vi "Build DashBoard Data.vi"(11 "Dashboard Enables":T3={"Analog Module 1"=[TRUE, TRUE, TRUE, TRUE, TRUE, TRUE, TRUE, TRUE], "Analog Module 2"=[FALSE, FALSE, FALSE, FALSE, FALSE, FALSE, FALSE, FALSE], "Digital Module 1"=TRUE, "Digital Module 2"=FALSE, "Solenoid Module"=TRUE}) -> ()   [LabVIEW 2012]
doc: "This VI builds data and sends it back to the dashboard PC program. By default it sends back the raw values for the first analog, digital, and solenoid module. Modify it to send back the data you want to view. Consider adding higher level data to the Dashboard Datatype.ctl and to this VI. Then update the Dashboard to display the data however you like.\n\nThis software is licensed. Open the labview\\readme\\WPI Robotics Library Open Source License.txt file for more information."
uses:
  DashboardEnable.ctl
  Dashboard Datatype.ctl
  <vilib>/Rock Robotics/WPI/DriverStation/WPI_DriverStationDigitalData.ctl
  <vilib>/Rock Robotics/SystemInterfaces/System/FPGA_SystemGet.vi
panel:
  out "Dashboard Data":T1
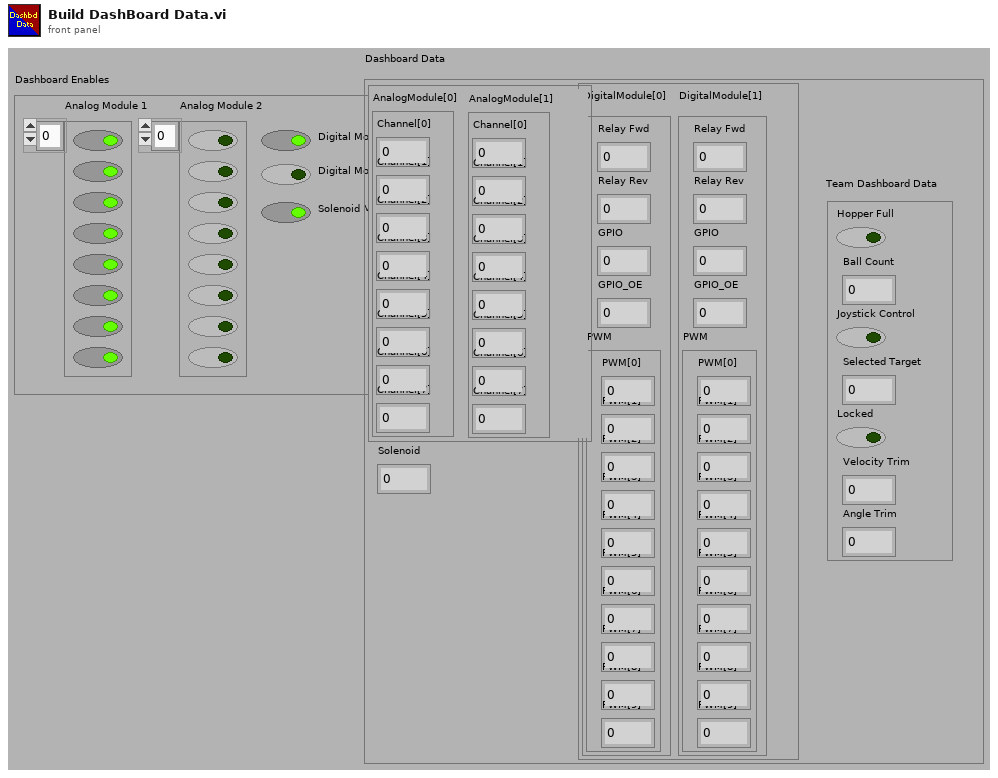
[diagram p1: front panel]
types:
  T1 = typedef "Dashboard Datatype.ctl" = cluster{cluster{"AnalogModule[0]":cluster{"Channel[0]":sgl, "Channel[1]":sgl, "Channel[2]":sgl, "Channel[3]":sgl, "Channel[4]":sgl, "Channel[5]":sgl, "Channel[6]":sgl, "Channel[7]":sgl}, "AnalogModule[1]":cluster{"Channel[0]":sgl, "Channel[1]":sgl, "Channel[2]":sgl, "Channel[3]":sgl, "Channel[4]":sgl, "Channel[5]":sgl, "Channel[6]":sgl, "Channel[7]":sgl}}, cluster{"DigitalModule[0]":T2, "DigitalModule[1]":T2}, "Solenoid":u8, "Team Dashboard Data":cluster{"Hopper Full":bool, "Ball Count":dbl, "Joystick Control":bool, "Selected Target":dbl, "Locked":bool, "Velocity Trim":dbl, "Angle Trim":dbl}}
  T2 = typedef "WPI_DriverStationDigitalData.ctl" = cluster{"Relay Fwd":u8, "Relay Rev":u8, "GPIO":u16, "GPIO_OE":u16, "PWM":cluster{"PWM[0]":u8, "PWM[1]":u8, "PWM[2]":u8, "PWM[3]":u8, "PWM[4]":u8, "PWM[5]":u8, "PWM[6]":u8, "PWM[7]":u8, "PWM[8]":u8, "PWM[9]":u8}}
  T3 = typedef "DashboardEnable.ctl" = cluster{"Analog Module 1":bool[], "Analog Module 2":bool[], "Digital Module 1":bool, "Digital Module 2":bool, "Solenoid Module":bool}
  T4 = cluster{"Hopper Full":bool, "Ball Count":dbl, "Joystick Control":bool, "Selected Target":dbl, "Locked":bool, "Velocity Trim":dbl, "Angle Trim":dbl}
  T5 = cluster{"AnalogModule[0]":cluster{"Channel[0]":sgl, "Channel[1]":sgl, "Channel[2]":sgl, "Channel[3]":sgl, "Channel[4]":sgl, "Channel[5]":sgl, "Channel[6]":sgl, "Channel[7]":sgl}, "AnalogModule[1]":cluster{"Channel[0]":sgl, "Channel[1]":sgl, "Channel[2]":sgl, "Channel[3]":sgl, "Channel[4]":sgl, "Channel[5]":sgl, "Channel[6]":sgl, "Channel[7]":sgl}}
  T6 = cluster{"Channel[0]":sgl, "Channel[1]":sgl, "Channel[2]":sgl, "Channel[3]":sgl, "Channel[4]":sgl, "Channel[5]":sgl, "Channel[6]":sgl, "Channel[7]":sgl}[]
  T7 = cluster{"Channel[0]":sgl, "Channel[1]":sgl, "Channel[2]":sgl, "Channel[3]":sgl, "Channel[4]":sgl, "Channel[5]":sgl, "Channel[6]":sgl, "Channel[7]":sgl}
  T8 = cluster{"AnalogModule[0][0]":sgl, "AnalogModule[0][1]":sgl, "AnalogModule[0][2]":sgl, "AnalogModule[0][3]":sgl, "AnalogModule[0][4]":sgl, "AnalogModule[0][5]":sgl, "AnalogModule[0][6]":sgl, "AnalogModule[0][7]":sgl}
  T9 = cluster{"[0]":cluster{"Channel[0]":sgl, "Channel[1]":sgl, "Channel[2]":sgl, "Channel[3]":sgl, "Channel[4]":sgl, "Channel[5]":sgl, "Channel[6]":sgl, "Channel[7]":sgl}, "[1]":cluster{"Channel[0]":sgl, "Channel[1]":sgl, "Channel[2]":sgl, "Channel[3]":sgl, "Channel[4]":sgl, "Channel[5]":sgl, "Channel[6]":sgl, "Channel[7]":sgl}}
  T10 = cluster{"DigitalModule[0]":T2, "DigitalModule[1]":T2}
  T11 = typedef "FPGA_DIODevRef.ctl" = cluster{"DevStatus":errorcluster, "Module":T12}
  T12 = typedef "FPGA_TypedefDigitalModule.ctl" = enum16{"Digital Module 1", "Digital Module 2"}
  T13 = cluster{"[0]":u8, "[1]":u8, "[2]":u8, "[3]":u8, "[4]":u8, "[5]":u8, "[6]":u8, "[7]":u8, "[8]":u8, "[9]":u8}
  T14 = typedef "FPGA_SolenoidDevRef.ctl" = cluster{"DevStatus":errorcluster, "Module":T15}
  T15 = typedef "FPGA_TypedefSolenoidModule.ctl" = enum16{"Solenoid Module 1", "Solenoid Module 2"}
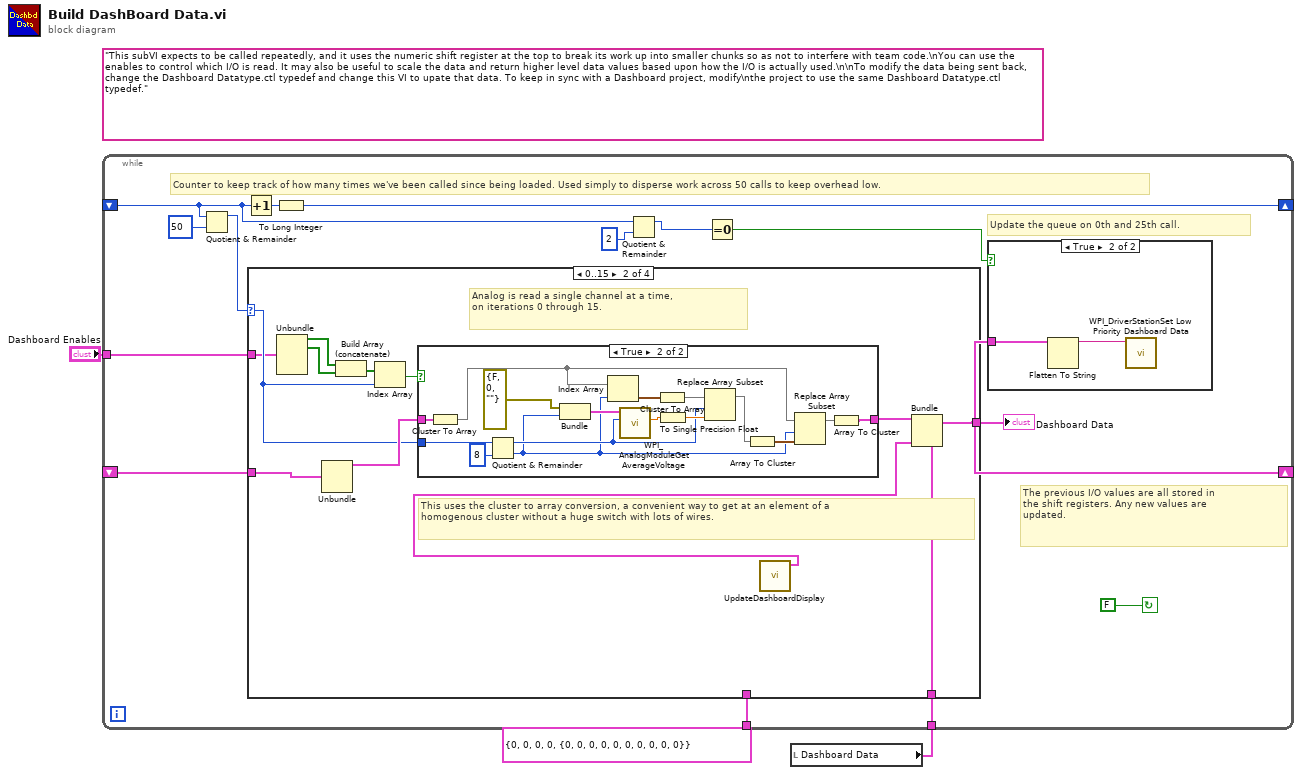
[diagram p0: block diagram]
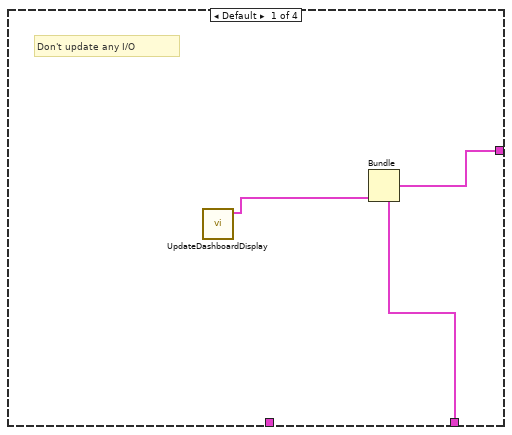
[diagram p3: hidden frame]
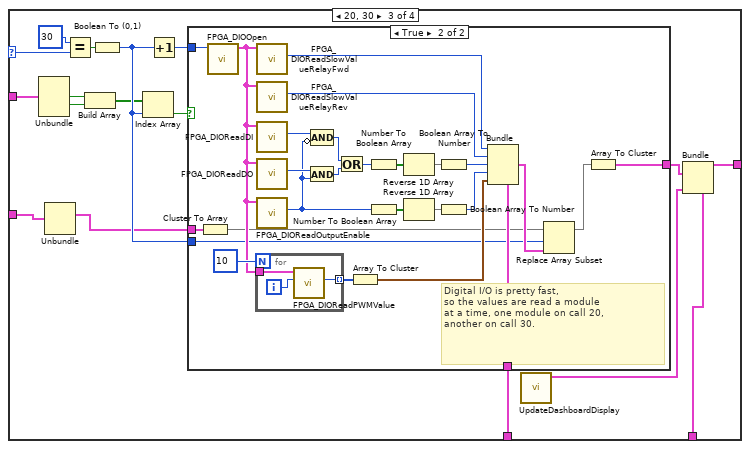
[diagram p5: hidden frame]
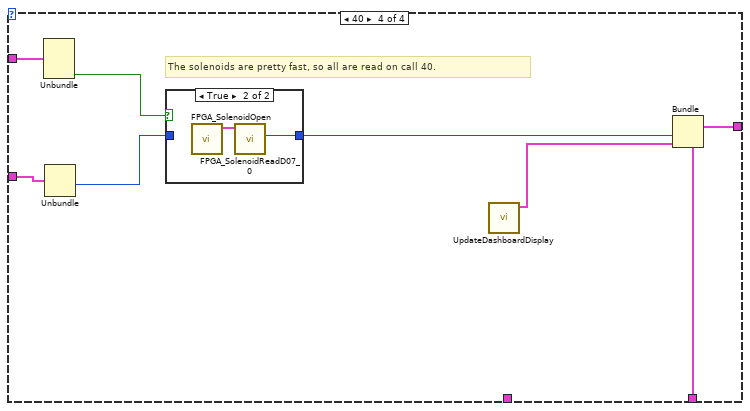
[diagram p7: hidden frame]
diagram:
  (unwired) "This subVI expects to be called repeatedly, and it uses the numeric shift register at the top to break its work up into smaller chunks so as not to interfere with team code.\nYou can use the enables to control which I/O is read. It may also be useful to scale the data and return higher level data values based upon how the I/O is actually used.\n\nTo modify the data being sent back, change the Dashboard Datatype.ctl typedef and change this VI to upate that data. To keep in sync with a Dashboard project, modify\nthe project to use the same Dashboard Datatype.ctl typedef."
  n1 = local read "Dashboard Data"() -> (w2:T1)
  n2 = while {
    shift-right: [w11] -> _
    shift-left: _ -> [w7]
    shift-right: [w8] -> _
    shift-left: _ -> [w15]
    tunnel: T2 {"Relay Fwd"=0, "Relay Rev"=0, "GPIO"=0, "GPIO_OE"=0, "PWM"={"PWM[0]"=0, "PWM[1]"=0, "PWM[2]"=0, "PWM[3]"=0, "PWM[4]"=0, "PWM[5]"=0, "PWM[6]"=0, "PWM[7]"=0, "PWM[8]"=0, "PWM[9]"=0}} ("DigitalModule[1]") -> [w14]
    tunnel: w2 -> [w10]
    tunnel: "Dashboard Enables" -> [w9]
    stop <- FALSE continue-if-true
    # "Counter to keep track of how many times we've been called since being loaded. Used simply to disperse work across 50 calls to keep overhead low."
    # "Update the queue on 0th and 25th call."
    # "The previous I/O values are all stored in\nthe shift registers. Any new values are\nupdated."
    n3 = Quotient & Remainder(x=w7, y=50) -> (x-y*floor(x/y)=w12:i32)  [unwired: 1 out]
    n4 = Increment(x=w7) -> (x+1=w17:i32)
    n5 = case shown="0..15" w12 {
      selector: w12 -> [_ w29 w62 _]
      tunnel: [w22 w25 w53 w103] -> w8
      tunnel: w15 -> [_ w24 w55 w105]
      tunnel: w14 -> [_ _ w68 _]
      tunnel: w10 -> [w21 w31 w54 w102]
      tunnel: w9 -> [_ w28 w60 w106]
      frame Default {
        # "Don't update any I/O"
        n6 = call "UpdateDashboardDisplay.vi"() -> ("Team Dashboard Data"=w20:T4)  [unwired: 11 in]
        n7 = Bundle(cluster=w21, "Team Dashboard Data"=w20) -> (w22:T1)  [unwired: 3 out]
      }
      frame 0..15 {
        # "This uses the cluster to array conversion, a convenient way to get at an element of a\nhomogenous cluster without a huge switch with lots of wires."
        # "Analog is read a single channel at a time,\non iterations 0 through 15."
        n8 = Unbundle(w28) -> ("Analog Module 1"=w27:bool[], "Analog Module 2"=w26:bool[])  [unwired: 3 out]
        n9 = Unbundle(w24) -> (w30:T5)  [unwired: 3 out]
        n10 = Build Array (concatenate)(w27, w26) -> (w33:bool[])
        n11 = Index Array(array=w33, index=w29) -> (element=w34:bool)
        n12 = case shown="True" w34 {
          tunnel: w29 -> [_ w42]
          tunnel: [w35 w39] -> w32
          tunnel: w30 -> [w35 w38]
          frame False {
          }
          frame True {
            n13 = Cluster To Array(cluster=w38) -> (array=w37:T6)
            n14 = Quotient & Remainder(x=w42, y=8) -> (x-y*floor(x/y)=w41:i32, floor(x/y)=w36:i32)
            n15 = Bundle("DevStatus"=errorcluster {"status"=FALSE, "code"=0, "source"=""}, w36) -> (w50:cluster{"DevStatus":errorcluster, i32})  [unwired: 1 out]
            n16 = Index Array(array=w37, index=w36) -> (element=w44:T7)
            n17 = call <vilib>:"WPI_AnalogModuleGetAverageVoltage.vi"("Channel"=w41, "AnalogModuleDevStatus"=w50) -> ("Average Voltage"=w47:dbl)  [unwired: 1 in, 8 out]
            n18 = Cluster To Array(cluster=w44) -> (array=w43:sgl[])
            n19 = To Single Precision Float(number=w47) -> (single precision float=w46:sgl)
            n20 = Replace Array Subset(array=w43, new element=w46, index=w41) -> (w45:sgl[])
            n21 = Array To Cluster(array=w45) -> (cluster=w49:T8)
            n22 = Replace Array Subset(array=w37, new element=w49, index=w36) -> (w40:T6)
            n23 = Array To Cluster(array=w40) -> (cluster=w39:T9)
          }
        }
        n24 = call "UpdateDashboardDisplay.vi"() -> ("Team Dashboard Data"=w23:T4)  [unwired: 11 in]
        n25 = Bundle(cluster=w31, w32, "Team Dashboard Data"=w23) -> (w25:T1)  [unwired: 2 out]
      }
      frame 20, 30 {
        n26 = Unbundle(w60) -> ("Digital Module 1"=w59:bool, "Digital Module 2"=w58:bool)  [unwired: 3 out]
        n27 = Unbundle(w55) -> (w57:T10)  [unwired: 3 out]
        n28 = Equal?(x=30, y=w62) -> (x = y?=w66:bool)
        n29 = Build Array(w59, w58) -> (w61:bool[])
        n30 = Boolean To (0,1)(Boolean=w66) -> (0, 1=w64:i16)
        n31 = Index Array(array=w61, index=w64) -> (element=w63:bool)
        n32 = Increment(x=w64) -> (x+1=w65:i16)
        n33 = case shown="True" w63 {
          tunnel: w68 -> [_ w77]
          tunnel: [w69 w70] -> w56
          tunnel: w65 -> [_ w75]
          tunnel: w64 -> [_ w74]
          tunnel: w57 -> [w69 w73]
          frame False {
          }
          frame True {
            # "Digital I/O is pretty fast,\nso the values are read a module\nat a time, one module on call 20,\nanother on call 30."
            n34 = Cluster To Array(cluster=w73) -> (array=w72:T2[])
            n35 = call <vilib>:"FPGA_DIOOpen.vi"("Module (Module 1)"=w75) -> ("DIODeviceRef"=w93:T11)  [unwired: 1 in, 9 out]
            n36 = for {
              N: 10 -> [_]
              tunnel: w93 -> [w98]
              tunnel: [w96] -> w94 mode=indexing
              i -> [w97]
              n37 = call <vilib>:"FPGA_DIOReadPWMValue.vi"("PWMChannel"=w97, "DIODeviceRef In"=w98) -> ("PWMValue"=w96:u8)  [unwired: 1 in, 8 out]
            }
            n38 = call <vilib>:"FPGA_DIOReadSlowValueRelayFwd.vi"("DIODeviceRef In"=w93) -> ("Relay Forward"=w86:u8)  [unwired: 1 in, 9 out]
            n39 = call <vilib>:"FPGA_DIOReadSlowValueRelayRev.vi"("DIODeviceRef In"=w93) -> ("Relay Reverse"=w87:u8)  [unwired: 1 in, 9 out]
            n40 = call <vilib>:"FPGA_DIOReadDI.vi"("DIODeviceRef In"=w93) -> ("DI"=w91:u16)  [unwired: 1 in, 9 out]
            n41 = call <vilib>:"FPGA_DIOReadDO.vi"("DIODeviceRef In"=w93) -> ("DO"=w90:u16)  [unwired: 1 in, 9 out]
            n42 = call <vilib>:"FPGA_DIOReadOutputEnable.vi"("DIODeviceRef In"=w93) -> ("OutputEnable"=w81:u16)  [unwired: 1 in, 9 out]
            n43 = And(x=w90, y=w81) -> (x .and. y?=w89:u16)
            n44 = Compound Arithmetic op=AND(w91, invert w81) -> (w88:u16)
            n45 = Or(x=w88, y=w89) -> (x .or. y?=w79:u16)
            n46 = Array To Cluster(array=w94) -> (cluster=w92:T13)
            n47 = Number To Boolean Array(number=w79) -> (Boolean array=w84:bool[])
            n48 = Number To Boolean Array(number=w81) -> (Boolean array=w83:bool[])
            n49 = Reverse 1D Array(array=w84) -> (reversed array=w85:bool[])
            n50 = Reverse 1D Array(array=w83) -> (reversed array=w82:bool[])
            n51 = Boolean Array To Number(Boolean array=w85) -> (number=w78:u32)
            n52 = Boolean Array To Number(Boolean array=w82) -> (number=w80:u32)
            n53 = Bundle(cluster=w77, "Relay Fwd"=w86, "Relay Rev"=w87, "GPIO"=w78, "GPIO_OE"=w80, "PWM"=w92) -> (w76:T2)
            n54 = Replace Array Subset(array=w72, new element=w76, index=w74) -> (w71:T2[])
            n55 = Array To Cluster(array=w71) -> (cluster=w70:cluster{"[0]":T2, "[1]":T2})
          }
        }
        n56 = call "UpdateDashboardDisplay.vi"() -> ("Team Dashboard Data"=w52:T4)  [unwired: 11 in]
        n57 = Bundle(cluster=w54, w56, "Team Dashboard Data"=w52) -> (w53:T1)  [unwired: 2 out]
      }
      frame 40 {
        # "The solenoids are pretty fast, so all are read on call 40."
        n58 = Unbundle(w106) -> ("Solenoid Module"=w100:bool)  [unwired: 4 out]
        n59 = Unbundle(w105) -> ("Solenoid"=w104:u8)  [unwired: 3 out]
        n60 = case shown="True" w100 {
          tunnel: [w107 w108] -> w101
          tunnel: w104 -> [w107 _]
          frame False {
          }
          frame True {
            n61 = call <vilib>:"FPGA_SolenoidOpen.vi"() -> ("SolenoidDevRef"=w109:T14)  [unwired: 2 in, 9 out]
            n62 = call <vilib>:"FPGA_SolenoidReadD07_0.vi"("SolenoidDevRef"=w109) -> ("DO7:0"=w108:u8)  [unwired: 1 in, 9 out]
          }
        }
        n63 = call "UpdateDashboardDisplay.vi"() -> ("Team Dashboard Data"=w99:T4)  [unwired: 11 in]
        n64 = Bundle(cluster=w102, "Solenoid"=w101, "Team Dashboard Data"=w99) -> (w103:T1)  [unwired: 2 out]
      }
    }
    "Dashboard Data" <- w8
    n65 = To Long Integer(number=w17) -> (32bit integer=w11:i32)
    n66 = Quotient & Remainder(x=w7, y=2) -> (x-y*floor(x/y)=w5:i32)  [unwired: 1 out]
    n67 = Equal To 0?(x=w5) -> (x = 0?=w4:bool)
    n68 = case shown="True" w4 {
      tunnel: w8 -> [_ w19]
      frame False {
      }
      frame True {
        n69 = Flatten To String(anything=w19) -> (data string=w18:string)  [unwired: 1 in, 4 out]
        n70 = call <vilib>:"WPI_DriverStationSet Low Priority Dashboard Data.vi"("User Data"=w18) -> ()  [unwired: 1 in, 10 out]
      }
    }
  }
